vi "WSVCAP SHL Host LL Core.vi"(0 "Message In":string, 11 "error in":errorcluster, 12 "Log (T)":bool=TRUE, 13 "Function":T3) -> (3 "System":T1={"Settings"={"FPGA Resource Name"="", "I2C Slave Address"=20, "I2C Clock Rate (Hz)"=50000.0, "SPI Clock Rate (Hz)"=50000.0, "RFFE Slave Address"=20, "RFFE Clock Rate (Hz)"=50000.0, "Simulate FPGA"=TRUE, "C1 Cap DAC Default"=165, "C2 Cap DAC Default"=134, "C3 Cap DAC Default"=150}, "FPGA Resource"="", "Online"=FALSE, "I2C Wait Ticks"=0, "SPI Wait Ticks"=0, "RFFE Wait Ticks"=0} {"Settings"."C3 Cap DAC Default" format="0x%02x"; "Settings"."C2 Cap DAC Default" format="0x%02x"; "Settings"."C1 Cap DAC Default" format="0x%02x"; "Settings"."RFFE Clock Rate (Hz)" format="%.0f Hz"; "Settings"."RFFE Slave Address" format="0x%02x"; "Settings"."I2C Clock Rate (Hz)" format="%.0f Hz"; "Settings"."SPI Clock Rate (Hz)" format="%.0f Hz"; "Settings"."I2C Slave Address" format="0x%02x"}, 4 "Message Out":string, 15 "error out":errorcluster)   [LabVIEW 2012]
uses:
  Type Defs/WSVCAP SHL Function Enum.ctl
  Type Defs/WSVCAP SHL Core System Cluster.ctl
  Type Defs/WSVCAP SHL I2C Settings Cluster.ctl
  user.lib/Utilities/Type Defs/MISC IO Choice Enum.ctl
  Type Defs/WSVCAP SHL Top Level Control Operation Enum.ctl
  Type Defs/WSVCAP SHL Top Level Control Enum.ctl
  Type Defs/WSVCAP SHL Manager Operation Enum.ctl
  user.lib/Configuration Files/Type Defs/CFG File Operation Enum.ctl
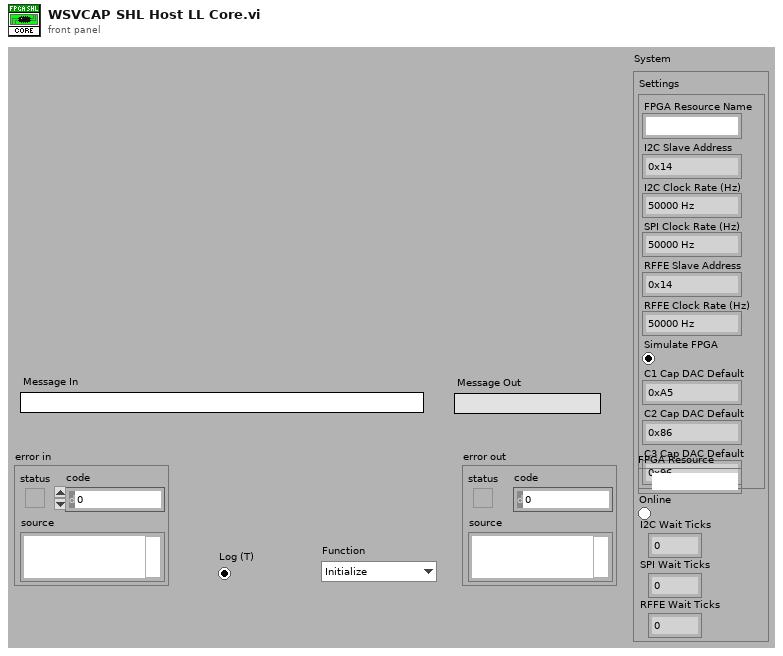
[diagram p1: front panel]
types:
  T1 = typedef "WSVCAP SHL Core System Cluster.ctl" = cluster{"Settings":T2, "FPGA Resource":tag, "Online":bool, "I2C Wait Ticks":u32, "SPI Wait Ticks":u32, "RFFE Wait Ticks":u32}
  T2 = typedef "WSVCAP SHL I2C Settings Cluster.ctl" = cluster{"FPGA Resource Name":string, "I2C Slave Address":u8, "I2C Clock Rate (Hz)":dbl, "SPI Clock Rate (Hz)":dbl, "RFFE Slave Address":u8, "RFFE Clock Rate (Hz)":dbl, "Simulate FPGA":bool, "C1 Cap DAC Default":u8, "C2 Cap DAC Default":u8, "C3 Cap DAC Default":u8}
  T3 = typedef "WSVCAP SHL Function Enum.ctl" = enum16{"Initialize", "Configure I2C", "Configure SPI", "Configure RFFE", "Write I2C", "Read I2C", "Write/Read SPI", "Start SPI Cycle", "Stop SPI Cycle", "Write RFFE", "Read RFFE", "Start RFFE Cycle", "Stop RFFE Cycle", "Get Status", "Close"}
  T4 = typedef "MISC IO Choice Enum.ctl" = enum16{"Read", "Write"}
  T5 = typedef "CFG File Operation Enum.ctl" = enum16{"Read", "Write", "Copy", "Edit"}
  T6 = typedef "WSVCAP SHL Manager Operation Enum.ctl" = enum16{"Initialize", "Close"}
  T7 = typedef "WSVCAP SHL Top Level Control Enum.ctl" = enum16{"Start", "Cmd", "Transaction", "Wait Ticks", "Socket Mask", "UUT Set", "Slave Address", "Sub Address", "Bytes to Write", "Bytes to Read", "Write Data", "Write Flag", "Read Data", "Read Flag", "Ack Read", "Read Status Flag", "Ack Read Status", "Status", "Cycle Count", "Stop Cycle", "Exit"}
  T8 = typedef "WSVCAP SHL Top Level Control Operation Enum.ctl" = enum16{"Initialize", "Set Control", "Read Control", "Close"}
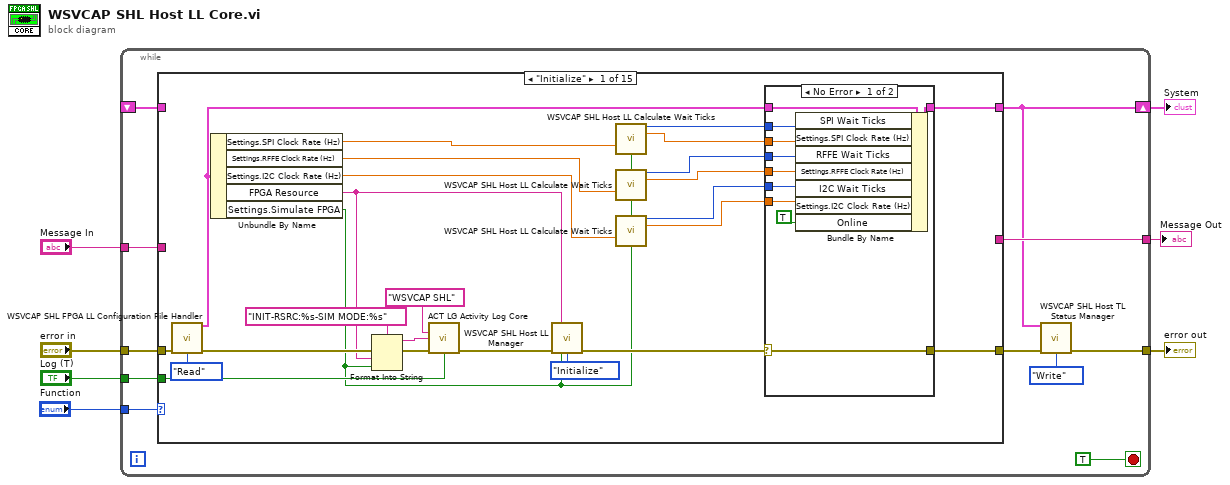
[diagram p0: block diagram]
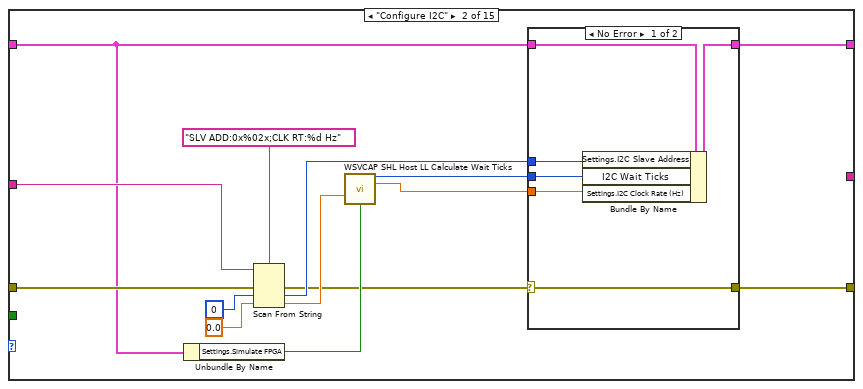
[diagram p3: hidden frame]
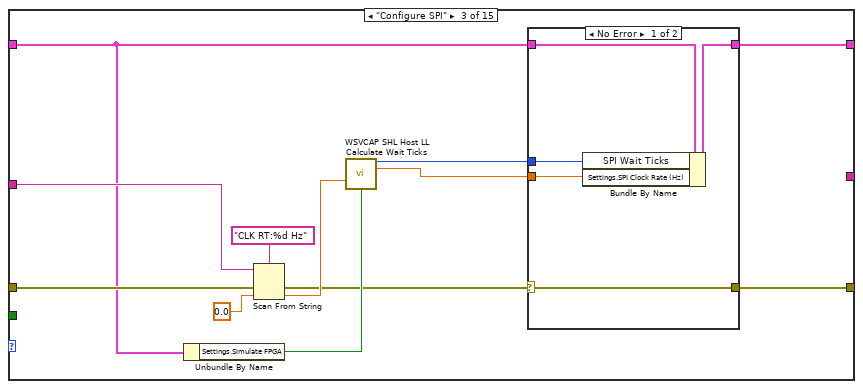
[diagram p5: hidden frame]
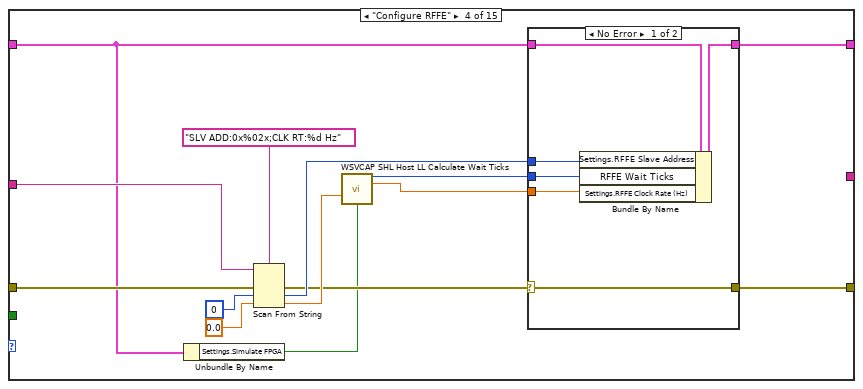
[diagram p7: hidden frame]
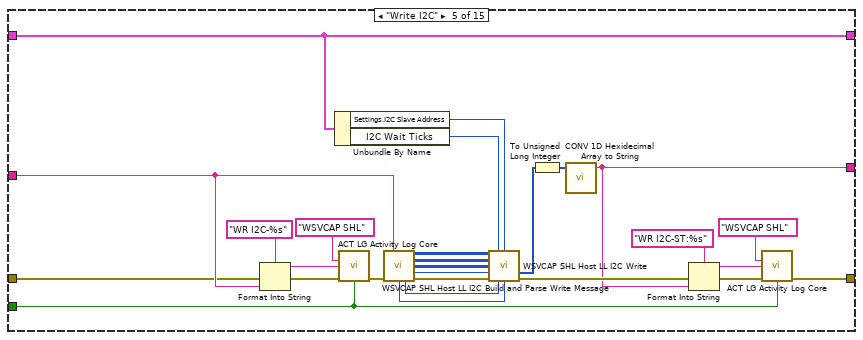
[diagram p9: hidden frame]
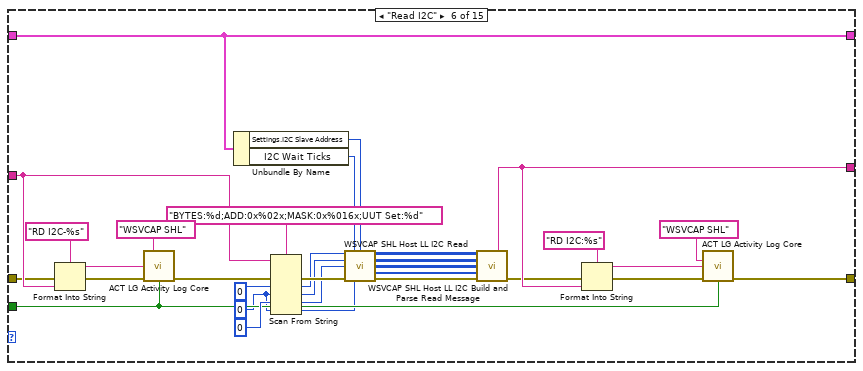
[diagram p10: hidden frame]
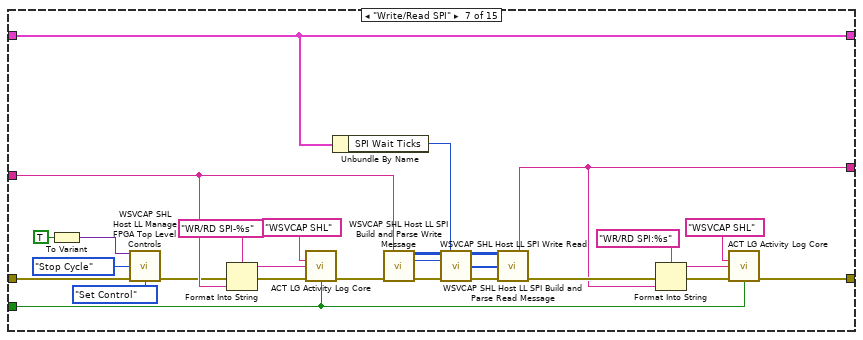
[diagram p11: hidden frame]
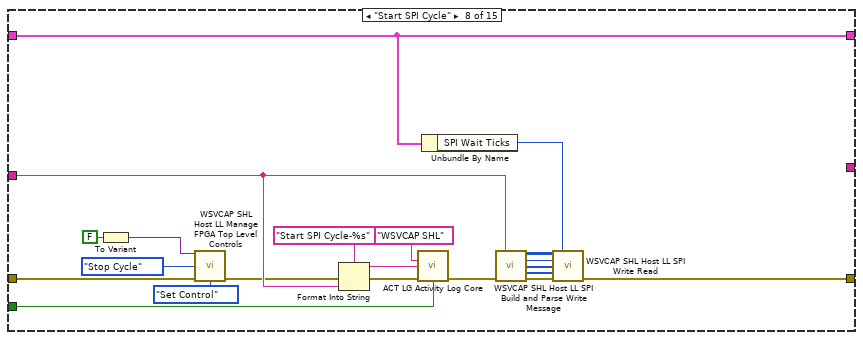
[diagram p12: hidden frame]
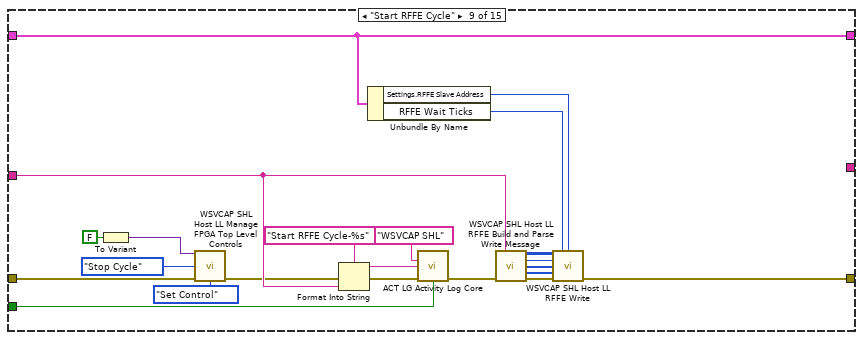
[diagram p13: hidden frame]
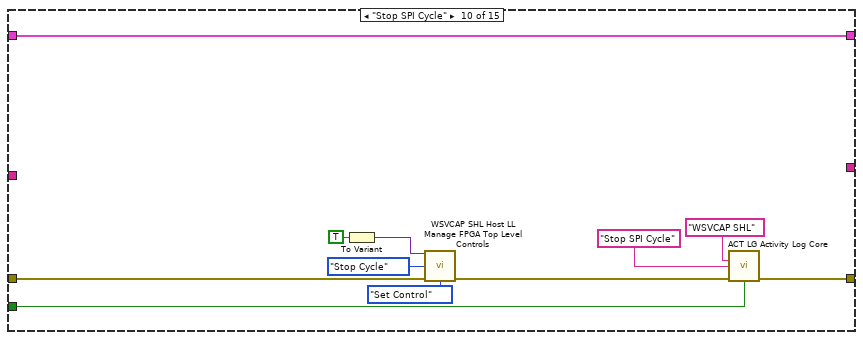
[diagram p14: hidden frame]
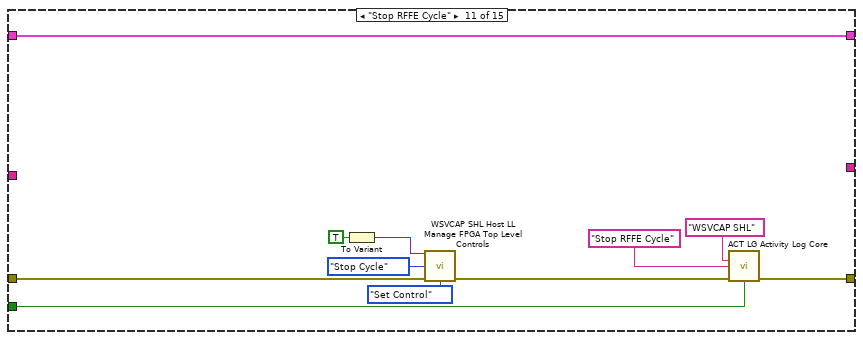
[diagram p15: hidden frame]
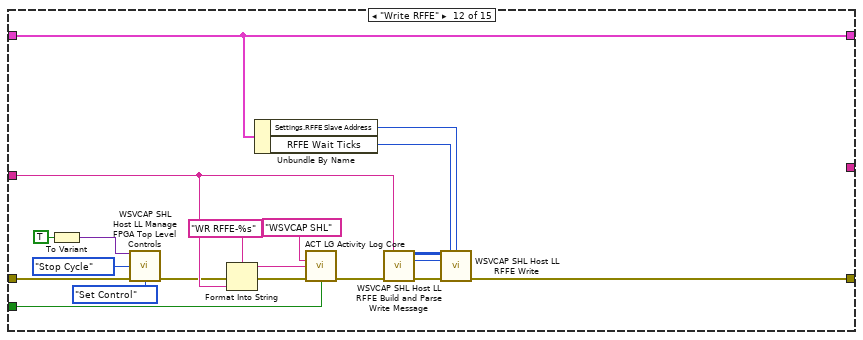
[diagram p16: hidden frame]
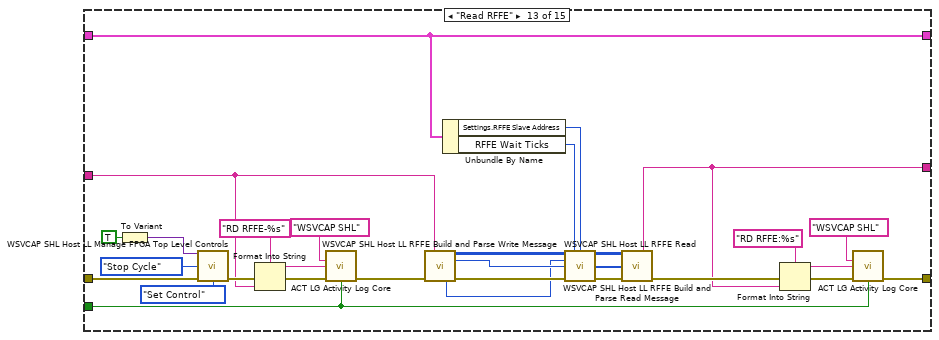
[diagram p17: hidden frame]
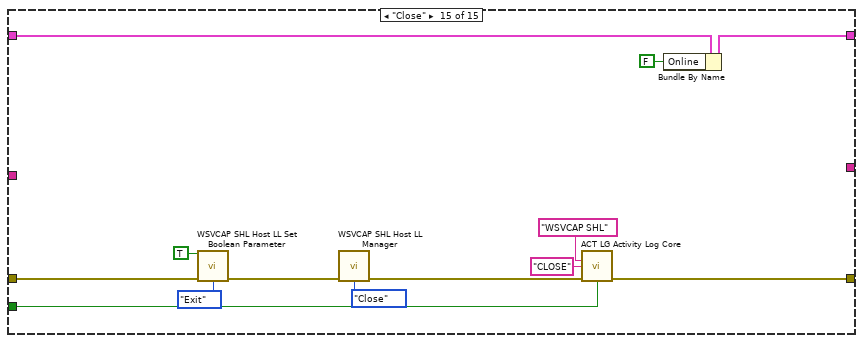
[diagram p19: hidden frame]
diagram:
  n1 = while {
    tunnel: "Function" -> [w17]
    tunnel: "error in" -> [w16]
    tunnel: "Message In" -> [w15]
    tunnel: [w11] -> w4
    shift-right: [w9] -> w3
    shift-left: _ -> [w14]
    tunnel: [w13] -> w2
    tunnel: "Log (T)" -> [w8]
    stop <- TRUE ("stop") stop-if-true
    n2 = case shown="\"Initialize\"" w17 {
      tunnel: w16 -> [w37 w67 w87 w108 w136 w159 w182 w209 w231 w250 w261 w277 w301 w321 w331]
      tunnel: w15 -> [_ w66 w86 w107 w137 w160 w188 w219 w241 _ _ w283 w294 _ _]
      tunnel: [w40 w68 w88 w109 w138 w156 w190 w217 w239 w257 w268 w272 w308 w321 w325] -> w12
      tunnel: [w41 w69 w89 w110 w124 w152 w179 w207 w229 w259 w270 w274 w299 w322 w334] -> w9
      tunnel: w14 -> [_ w62 w84 w103 w124 w152 w179 w207 w229 w259 w270 w274 w299 w322 w329]
      tunnel: [_ _ _ _ w128 w161 w189 _ _ _ _ _ w307 _ _] -> w13
      tunnel: w8 -> [w28 _ _ _ w125 w153 w187 w218 w240 w256 w267 w282 w306 _ w323]
      frame "Initialize" {
        n3 = call "WSVCAP SHL FPGA LL Configuration File Handler.vi"("Error In (no error)"=w37, "Operation"=CFG_File_Operation_Enum."Read") -> ("Object Cluster Out"=w42:T1, "Error Out"=w34:errorcluster)  [unwired: 11 in, 1 out]
        n4 = Unbundle By Name(w42) -> ("Settings.SPI Clock Rate (Hz)"=w22:dbl, "Settings.RFFE Clock Rate (Hz)"=w26:dbl, "Settings.I2C Clock Rate (Hz)"=w30:dbl, "FPGA Resource"=w31:tag, "Settings.Simulate FPGA"=w19:bool)
        n5 = Format Into String(format string="INIT-RSRC:%s-SIM MODE:%s", error in=w34, w31, w19) -> (resulting string=w35:string, error out=w33:errorcluster)  [unwired: 1 in]
        n6 = call "ACT LG Activity Log Core.vi"("Source"="WSVCAP SHL", "Log Line"=w35, "Error In (no error)"=w33, "Log (T)"=w28) -> ("Error Out"=w36:errorcluster)  [unwired: 10 in, 1 out]
        n7 = call "WSVCAP SHL Host LL Manager.vi"("FPGA Resource (Init Only)"=w31, "error in (no error)"=w36, "Simulate FPGA (Init Only)"=w19, "Operation"=WSVCAP_SHL_Manager_Operation_Enum."Initialize") -> ("error out"=w23:errorcluster)  [unwired: 11 in]
        n8 = call "WSVCAP SHL Host LL Calculate Wait Ticks.vi"("Clock Rate (Hz)"=w22, "Simulate FPGA"=w19) -> ("Wait Ticks"=w21:u32, "Actual Rate (Hz)"=w20:dbl)  [unwired: 12 in]
        n9 = call "WSVCAP SHL Host LL Calculate Wait Ticks.vi"("Clock Rate (Hz)"=w26, "Simulate FPGA"=w19) -> ("Wait Ticks"=w25:u32, "Actual Rate (Hz)"=w24:dbl)  [unwired: 12 in]
        n10 = call "WSVCAP SHL Host LL Calculate Wait Ticks.vi"("Clock Rate (Hz)"=w30, "Simulate FPGA"=w19) -> ("Wait Ticks"=w27:u32, "Actual Rate (Hz)"=w39:dbl)  [unwired: 12 in]
        n11 = case shown="No Error" w23 {
          selector: w23 -> [w51 w54]
          tunnel: w42 -> [w53 w55]
          tunnel: [w52 w55] -> w41
          tunnel: [w51 w54] -> w40
          tunnel: w39 -> [w50 _]
          tunnel: w27 -> [w48 _]
          tunnel: w25 -> [w47 _]
          tunnel: w24 -> [w46 _]
          tunnel: w21 -> [w45 _]
          tunnel: w20 -> [w44 _]
          frame No Error {
            n12 = Bundle By Name(cluster=w53, "SPI Wait Ticks"=w45, "Settings.SPI Clock Rate (Hz)"=w44, "RFFE Wait Ticks"=w47, "Settings.RFFE Clock Rate (Hz)"=w46, "I2C Wait Ticks"=w48, "Settings.I2C Clock Rate (Hz)"=w50, "Online"=TRUE) -> (w52:T1)
          }
          frame Error {
          }
        }
      }
      frame "Configure I2C" {
        n13 = Unbundle By Name(w62) -> ("Settings.Simulate FPGA"=w61:bool)
        n14 = Scan From String(format string="SLV ADD:0x%02x;CLK RT:%d Hz", input string=w66, error in=w67, default 1=u8 0 ("I2C_Slave Address"), default 2=0.0 ("Clock Rate (Hz)")) -> (error out=w56:errorcluster, output 1=w63:u8, output 2=w59:dbl)  [unwired: 1 in, 2 out]
        n15 = call "WSVCAP SHL Host LL Calculate Wait Ticks.vi"("Clock Rate (Hz)"=w59, "Simulate FPGA"=w61) -> ("Wait Ticks"=w57:u32, "Actual Rate (Hz)"=w58:dbl)  [unwired: 12 in]
        n16 = case shown="No Error" w56 {
          selector: w56 -> [w73 w76]
          tunnel: w62 -> [w75 w77]
          tunnel: [w74 w77] -> w69
          tunnel: [w73 w76] -> w68
          tunnel: w63 -> [w72 _]
          tunnel: w58 -> [w71 _]
          tunnel: w57 -> [w70 _]
          frame No Error {
            n17 = Bundle By Name(cluster=w75, "Settings.I2C Slave Address"=w72, "I2C Wait Ticks"=w70, "Settings.I2C Clock Rate (Hz)"=w71) -> (w74:T1)
          }
          frame Error {
          }
        }
      }
      frame "Configure SPI" {
        n18 = Unbundle By Name(w84) -> ("Settings.Simulate FPGA"=w79:bool)
        n19 = Scan From String(format string="CLK RT:%d Hz", input string=w86, error in=w87, default 1=0.0 ("Clock Rate (Hz)")) -> (error out=w78:errorcluster, output 1=w82:dbl)  [unwired: 1 in, 2 out]
        n20 = call "WSVCAP SHL Host LL Calculate Wait Ticks.vi"("Clock Rate (Hz)"=w82, "Simulate FPGA"=w79) -> ("Wait Ticks"=w81:u32, "Actual Rate (Hz)"=w80:dbl)  [unwired: 12 in]
        n21 = case shown="No Error" w78 {
          selector: w78 -> [w92 w95]
          tunnel: w84 -> [w94 w96]
          tunnel: [w93 w96] -> w89
          tunnel: [w92 w95] -> w88
          tunnel: w80 -> [w91 _]
          tunnel: w81 -> [w90 _]
          frame No Error {
            n22 = Bundle By Name(cluster=w94, "SPI Wait Ticks"=w90, "Settings.SPI Clock Rate (Hz)"=w91) -> (w93:T1)
          }
          frame Error {
          }
        }
      }
      frame "Configure RFFE" {
        n23 = Unbundle By Name(w103) -> ("Settings.Simulate FPGA"=w97:bool)
        n24 = Scan From String(format string="SLV ADD:0x%02x;CLK RT:%d Hz", input string=w107, error in=w108, default 1=u8 0 ("I2C_Slave Address"), default 2=0.0 ("Clock Rate (Hz)")) -> (error out=w98:errorcluster, output 1=w104:u8, output 2=w101:dbl)  [unwired: 1 in, 2 out]
        n25 = call "WSVCAP SHL Host LL Calculate Wait Ticks.vi"("Clock Rate (Hz)"=w101, "Simulate FPGA"=w97) -> ("Wait Ticks"=w100:u32, "Actual Rate (Hz)"=w99:dbl)  [unwired: 12 in]
        n26 = case shown="No Error" w98 {
          selector: w98 -> [w114 w117]
          tunnel: w103 -> [w116 w118]
          tunnel: [w115 w118] -> w110
          tunnel: [w114 w117] -> w109
          tunnel: w104 -> [w113 _]
          tunnel: w99 -> [w112 _]
          tunnel: w100 -> [w111 _]
          frame No Error {
            n27 = Bundle By Name(cluster=w116, "Settings.RFFE Slave Address"=w113, "RFFE Wait Ticks"=w111, "Settings.RFFE Clock Rate (Hz)"=w112) -> (w115:T1)
          }
          frame Error {
          }
        }
      }
      frame "Write I2C" {
        n28 = Format Into String(format string="WR I2C-%s", error in=w136, w137) -> (resulting string=w133:string, error out=w135:errorcluster)  [unwired: 1 in]
        n29 = Unbundle By Name(w124) -> ("Settings.I2C Slave Address"=w120:u8, "I2C Wait Ticks"=w123:u32)
        n30 = call "ACT LG Activity Log Core.vi"("Source"="WSVCAP SHL", "Log Line"=w133, "Error In (no error)"=w135, "Log (T)"=w125) -> ("Error Out"=w140:errorcluster)  [unwired: 10 in, 1 out]
        n31 = call "WSVCAP SHL Host LL I2C Build and Parse Write Message.vi"("Message In"=w137, "error in"=w140) -> ("C1 Write Data Out [DUT Ordered]"=w144:u8[][], "C2 Write Data Out [DUT Ordered]"=w142:u8[][], "C3 Write Data Out [DUT Ordered]"=w122:u8[][], "Socket Mask [U64] Out"=w143:u64, "UUT Set (0/1) Out"=w119:u8, "Sub Address Out"=w121:u8, "error out"=w145:errorcluster)  [unwired: 6 in, 1 out]
        n32 = call "WSVCAP SHL Host LL I2C Write.vi"("C1 Data Out [DUT Ordered]"=w144, "Wait Ticks"=w123, "Slave Address"=w120, "C2 Data Out [DUT Ordered]"=w142, "C3 Data Out [DUT Ordered]"=w122, "Socket Mask [U64]"=w143, "error in"=w145, "Sub Address"=w121, "UUT Set (0/1)"=w119) -> ("Status"=w130:u8[], "error out"=w132:errorcluster)  [unwired: 5 in]
        n33 = To Unsigned Long Integer(number=w130) -> (unsigned 32bit integer=w129:u32[])
        n34 = call "CONV 1D Hexidecimal Array to String.vi"("1-D Hexidecimal"=w129) -> ("String"=w128:string)  [unwired: 8 in]
        n35 = Format Into String(format string="WR I2C-ST:%s", error in=w132, w128) -> (resulting string=w126:string, error out=w131:errorcluster)  [unwired: 1 in]
        n36 = call "ACT LG Activity Log Core.vi"("Source"="WSVCAP SHL", "Log Line"=w126, "Error In (no error)"=w131, "Log (T)"=w125) -> ("Error Out"=w138:errorcluster)  [unwired: 10 in, 1 out]
      }
      frame "Read I2C" {
        w147 = u8 0 ("Sub Address [U8]")
        n37 = Format Into String(format string="RD I2C-%s", error in=w159, w160) -> (resulting string=w165:string, error out=w167:errorcluster)  [unwired: 1 in]
        n38 = call "ACT LG Activity Log Core.vi"("Source"="WSVCAP SHL", "Log Line"=w165, "Error In (no error)"=w167, "Log (T)"=w153) -> ("Error Out"=w158:errorcluster)  [unwired: 10 in, 1 out]
        n39 = Unbundle By Name(w152) -> ("Settings.I2C Slave Address"=w148:u8, "I2C Wait Ticks"=w151:u32)
        n40 = Scan From String(format string="BYTES:%d;ADD:0x%02x;MASK:0x%016x;UUT Set:%d", input string=w160, error in=w158, default 1=u8 0 ("Bytes to Read"), default 2=w147, default 3=u64 0 ("Socket Mask [U32]"), default 4=w147) -> (error out=w177:errorcluster, output 1=w174:u8, output 2=w172:u8, output 3=w173:u64, output 4=w146:u8)  [unwired: 1 in, 2 out]
        n41 = call "WSVCAP SHL Host LL I2C Read.vi"("Bytes to Read"=w174, "Wait Ticks"=w151, "Slave Address"=w148, "Sub Address [U8]"=w172, "Socket Mask [U64]"=w173, "error in"=w177, "UUT Set (0/1)"=w146) -> ("C1:1-18 Read Data [DUT Ordered]"=w170:u8[][], "C2:1-18 Read Data [DUT Ordered]"=w169:u8[][], "C3:1-18 Read Data [DUT Ordered]"=w150:u8[][], "Status"=w149:u8[], "error out"=w171:errorcluster)  [unwired: 4 in]
        n42 = call "WSVCAP SHL Host LL I2C Build and Parse Read Message.vi"("C1 Read Data In"=w170, "C2 Read Data"=w169, "C3 Read Data"=w150, "Status In"=w149, "error in"=w171) -> ("Message Out"=w161:string, "error out"=w157:errorcluster)  [unwired: 5 in, 4 out]
        n43 = Format Into String(format string="RD I2C:%s", error in=w157, w161) -> (resulting string=w162:string, error out=w164:errorcluster)  [unwired: 1 in]
        n44 = call "ACT LG Activity Log Core.vi"("Source"="WSVCAP SHL", "Log Line"=w162, "Error In (no error)"=w164, "Log (T)"=w153) -> ("Error Out"=w156:errorcluster)  [unwired: 10 in, 1 out]
      }
      frame "Write/Read SPI" {
        n45 = To Variant(anything=TRUE ("Cycle (F:Write/Read - T:Write Only - No Read)")) -> (Variant=w184:variant)
        n46 = call "WSVCAP SHL Host LL Manage FPGA Top Level Controls.vi"("Value In"=w184, "FPGA Top Level Control"=WSVCAP_SHL_Top_Level_Control_Enum."Stop Cycle", "error in (no error)"=w182, "Operation"=WSVCAP_SHL_Top_Level_Control_Operation_Enum."Set Control") -> ("error out"=w181:errorcluster)  [unwired: 10 in, 1 out]
        n47 = Format Into String(format string="WR/RD SPI-%s", error in=w181, w188) -> (resulting string=w196:string, error out=w198:errorcluster)  [unwired: 1 in]
        n48 = call "ACT LG Activity Log Core.vi"("Source"="WSVCAP SHL", "Log Line"=w196, "Error In (no error)"=w198, "Log (T)"=w187) -> ("Error Out"=w192:errorcluster)  [unwired: 10 in, 1 out]
        n49 = Unbundle By Name(w179) -> ("SPI Wait Ticks"=w178:u32)
        n50 = call "WSVCAP SHL Host LL SPI Build and Parse Write Message.vi"("Message In"=w188, "error in"=w192) -> ("Write Data Out [DUT Ordered]"=w204:u8[][], "Socket Mask [U16] Out"=w180:u16, "error out"=w205:errorcluster)  [unwired: 8 in, 3 out]
        n51 = call "WSVCAP SHL Host LL SPI Write Read.vi"("SPI Data [DUT Ordered]"=w204, "Wait Ticks"=w178, "Socket Mask"=w180, "error in"=w205) -> ("SPI Read Data [DUT Ordered]"=w202:u8[][], "Status"=w201:u8[], "error out"=w203:errorcluster)  [unwired: 9 in]
        n52 = call "WSVCAP SHL Host LL SPI Build and Parse Read Message.vi"("Write Data In"=w202, "Status In"=w201, "error in"=w203) -> ("Message Out"=w189:string, "error out"=w191:errorcluster)  [unwired: 9 in, 2 out]
        n53 = Format Into String(format string="WR/RD SPI:%s", error in=w191, w189) -> (resulting string=w193:string, error out=w195:errorcluster)  [unwired: 1 in]
        n54 = call "ACT LG Activity Log Core.vi"("Source"="WSVCAP SHL", "Log Line"=w193, "Error In (no error)"=w195, "Log (T)"=w187) -> ("Error Out"=w190:errorcluster)  [unwired: 10 in, 1 out]
      }
      frame "Start SPI Cycle" {
        n55 = To Variant(anything=FALSE ("Cycle (F:Write/Read - T:Write Only - No Read)")) -> (Variant=w214:variant)
        n56 = call "WSVCAP SHL Host LL Manage FPGA Top Level Controls.vi"("Value In"=w214, "FPGA Top Level Control"=WSVCAP_SHL_Top_Level_Control_Enum."Stop Cycle", "error in (no error)"=w209, "Operation"=WSVCAP_SHL_Top_Level_Control_Operation_Enum."Set Control") -> ("error out"=w208:errorcluster)  [unwired: 10 in, 1 out]
        n57 = Format Into String(format string="Start SPI Cycle-%s", error in=w208, w219) -> (resulting string=w221:string, error out=w223:errorcluster)  [unwired: 1 in]
        n58 = call "ACT LG Activity Log Core.vi"("Source"="WSVCAP SHL", "Log Line"=w221, "Error In (no error)"=w223, "Log (T)"=w218) -> ("Error Out"=w220:errorcluster)  [unwired: 10 in, 1 out]
        n59 = Unbundle By Name(w207) -> ("SPI Wait Ticks"=w206:u32)
        n60 = call "WSVCAP SHL Host LL SPI Build and Parse Write Message.vi"("Message In"=w219, "error in"=w220) -> ("Write Data Out [DUT Ordered]"=w225:u8[][], "Socket Mask [U16] Out"=w212:u16, "Cycle CMD Lengths Out (bits)"=w211:u8[], "Cycle CMD Delay Out (ticks)"=w210:u32[], "error out"=w226:errorcluster)  [unwired: 8 in, 1 out]
        n61 = call "WSVCAP SHL Host LL SPI Write Read.vi"("SPI Data [DUT Ordered]"=w225, "Wait Ticks"=w206, "Socket Mask"=w212, "Cycle CMD Lengths Out (bits)"=w211, "Cycle CMD Delay Out (ticks)"=w210, "error in"=w226) -> ("error out"=w217:errorcluster)  [unwired: 7 in, 2 out]
      }
      frame "Start RFFE Cycle" {
        n62 = To Variant(anything=FALSE ("Cycle (F:Write/Read - T:Write Only - No Read)")) -> (Variant=w236:variant)
        n63 = call "WSVCAP SHL Host LL Manage FPGA Top Level Controls.vi"("Value In"=w236, "FPGA Top Level Control"=WSVCAP_SHL_Top_Level_Control_Enum."Stop Cycle", "error in (no error)"=w231, "Operation"=WSVCAP_SHL_Top_Level_Control_Operation_Enum."Set Control") -> ("error out"=w230:errorcluster)  [unwired: 10 in, 1 out]
        n64 = Format Into String(format string="Start RFFE Cycle-%s", error in=w230, w241) -> (resulting string=w243:string, error out=w245:errorcluster)  [unwired: 1 in]
        n65 = Unbundle By Name(w229) -> ("Settings.RFFE Slave Address"=w227:u8, "RFFE Wait Ticks"=w228:u32)
        n66 = call "ACT LG Activity Log Core.vi"("Source"="WSVCAP SHL", "Log Line"=w243, "Error In (no error)"=w245, "Log (T)"=w240) -> ("Error Out"=w242:errorcluster)  [unwired: 10 in, 1 out]
        n67 = call "WSVCAP SHL Host LL RFFE Build and Parse Write Message.vi"("Message In"=w241, "error in"=w242) -> ("Write Data Out [DUT Ordered]"=w247:u8[][], "Socket Mask [U16] Out"=w234:u64, "Cycle CMD Lengths Out (bits)"=w233:u8[], "Cycle CMD Delay Out (ticks)"=w232:u32[], "error out"=w248:errorcluster)  [unwired: 7 in, 2 out]
        n68 = call "WSVCAP SHL Host LL RFFE Write.vi"("RTFFE Data [DUT Ordered]"=w247, "Wait Ticks"=w228, "Slave Address"=w227, "Socket Mask"=w234, "Cycle CMD Lengths Out (bits)"=w233, "Cycle CMD Delay Out (ticks)"=w232, "error in"=w248) -> ("error out"=w239:errorcluster)  [unwired: 7 in, 1 out]
      }
      frame "Stop SPI Cycle" {
        n69 = To Variant(anything=TRUE ("Cycle (F:Write/Read - T:Write Only - No Read)")) -> (Variant=w252:variant)
        n70 = call "WSVCAP SHL Host LL Manage FPGA Top Level Controls.vi"("Value In"=w252, "FPGA Top Level Control"=WSVCAP_SHL_Top_Level_Control_Enum."Stop Cycle", "error in (no error)"=w250, "Operation"=WSVCAP_SHL_Top_Level_Control_Operation_Enum."Set Control") -> ("error out"=w249:errorcluster)  [unwired: 10 in, 1 out]
        n71 = call "ACT LG Activity Log Core.vi"("Source"="WSVCAP SHL", "Log Line"="Stop SPI Cycle" ("format string"), "Error In (no error)"=w249, "Log (T)"=w256) -> ("Error Out"=w257:errorcluster)  [unwired: 10 in, 1 out]
      }
      frame "Stop RFFE Cycle" {
        n72 = To Variant(anything=TRUE ("Cycle (F:Write/Read - T:Write Only - No Read)")) -> (Variant=w263:variant)
        n73 = call "WSVCAP SHL Host LL Manage FPGA Top Level Controls.vi"("Value In"=w263, "FPGA Top Level Control"=WSVCAP_SHL_Top_Level_Control_Enum."Stop Cycle", "error in (no error)"=w261, "Operation"=WSVCAP_SHL_Top_Level_Control_Operation_Enum."Set Control") -> ("error out"=w260:errorcluster)  [unwired: 10 in, 1 out]
        n74 = call "ACT LG Activity Log Core.vi"("Source"="WSVCAP SHL", "Log Line"="Stop RFFE Cycle" ("format string"), "Error In (no error)"=w260, "Log (T)"=w267) -> ("Error Out"=w268:errorcluster)  [unwired: 10 in, 1 out]
      }
      frame "Write RFFE" {
        n75 = To Variant(anything=TRUE ("Cycle (F:Write/Read - T:Write Only - No Read)")) -> (Variant=w279:variant)
        n76 = call "WSVCAP SHL Host LL Manage FPGA Top Level Controls.vi"("Value In"=w279, "FPGA Top Level Control"=WSVCAP_SHL_Top_Level_Control_Enum."Stop Cycle", "error in (no error)"=w277, "Operation"=WSVCAP_SHL_Top_Level_Control_Operation_Enum."Set Control") -> ("error out"=w276:errorcluster)  [unwired: 10 in, 1 out]
        n77 = Format Into String(format string="WR RFFE-%s", error in=w276, w283) -> (resulting string=w285:string, error out=w287:errorcluster)  [unwired: 1 in]
        n78 = Unbundle By Name(w274) -> ("Settings.RFFE Slave Address"=w271:u8, "RFFE Wait Ticks"=w273:u32)
        n79 = call "ACT LG Activity Log Core.vi"("Source"="WSVCAP SHL", "Log Line"=w285, "Error In (no error)"=w287, "Log (T)"=w282) -> ("Error Out"=w284:errorcluster)  [unwired: 10 in, 1 out]
        n80 = call "WSVCAP SHL Host LL RFFE Build and Parse Write Message.vi"("Message In"=w283, "error in"=w284) -> ("Write Data Out [DUT Ordered]"=w289:u8[][], "Socket Mask [U16] Out"=w275:u64, "error out"=w290:errorcluster)  [unwired: 7 in, 4 out]
        n81 = call "WSVCAP SHL Host LL RFFE Write.vi"("RTFFE Data [DUT Ordered]"=w289, "Wait Ticks"=w273, "Slave Address"=w271, "Socket Mask"=w275, "error in"=w290) -> ("error out"=w272:errorcluster)  [unwired: 9 in, 1 out]
      }
      frame "Read RFFE" {
        n82 = To Variant(anything=TRUE ("Cycle (F:Write/Read - T:Write Only - No Read)")) -> (Variant=w303:variant)
        n83 = call "WSVCAP SHL Host LL Manage FPGA Top Level Controls.vi"("Value In"=w303, "FPGA Top Level Control"=WSVCAP_SHL_Top_Level_Control_Enum."Stop Cycle", "error in (no error)"=w301, "Operation"=WSVCAP_SHL_Top_Level_Control_Operation_Enum."Set Control") -> ("error out"=w300:errorcluster)  [unwired: 10 in, 1 out]
        n84 = Format Into String(format string="RD RFFE-%s", error in=w300, w294) -> (resulting string=w313:string, error out=w315:errorcluster)  [unwired: 1 in]
        n85 = call "ACT LG Activity Log Core.vi"("Source"="WSVCAP SHL", "Log Line"=w313, "Error In (no error)"=w315, "Log (T)"=w306) -> ("Error Out"=w296:errorcluster)  [unwired: 10 in, 1 out]
        n86 = call "WSVCAP SHL Host LL RFFE Build and Parse Write Message.vi"("Message In"=w294, "error in"=w296) -> ("Write Data Out [DUT Ordered]"=w293:u8[][], "Socket Mask [U16] Out"=w292:u64, "Byte Count"=w291:u8, "error out"=w295:errorcluster)  [unwired: 7 in, 3 out]
        n87 = Unbundle By Name(w299) -> ("Settings.RFFE Slave Address"=w297:u8, "RFFE Wait Ticks"=w298:u32)
        n88 = call "WSVCAP SHL Host LL RFFE Read.vi"("RFFE Data [DUT Ordered]"=w293, "Wait Ticks"=w298, "Slave Address"=w297, "Bytes to Read"=w291, "Socket Mask [U64]"=w292, "error in"=w295) -> ("RFFE Read Data [DUT Ordered]"=w319:u8[][], "Status"=w318:u8[], "error out"=w320:errorcluster)  [unwired: 7 in]
        n89 = call "WSVCAP SHL Host LL RFFE Build and Parse Read Message.vi"("Write Data In"=w319, "Status In"=w318, "error in"=w320) -> ("Message Out"=w307:string, "error out"=w309:errorcluster)  [unwired: 9 in, 2 out]
        n90 = Format Into String(format string="RD RFFE:%s", error in=w309, w307) -> (resulting string=w310:string, error out=w312:errorcluster)  [unwired: 1 in]
        n91 = call "ACT LG Activity Log Core.vi"("Source"="WSVCAP SHL", "Log Line"=w310, "Error In (no error)"=w312, "Log (T)"=w306) -> ("Error Out"=w308:errorcluster)  [unwired: 10 in, 1 out]
      }
      frame "Get Status" {
      }
      frame "Close" {
        n92 = call "WSVCAP SHL Host LL Set Boolean Parameter.vi"("Boolean In"=TRUE ("Start"), "error in (no error)"=w331, "FPGA Top Level Control"=WSVCAP_SHL_Top_Level_Control_Enum."Exit") -> ("error out"=w330:errorcluster)  [unwired: 12 in]
        n93 = call "WSVCAP SHL Host LL Manager.vi"("error in (no error)"=w330, "Operation"=WSVCAP_SHL_Manager_Operation_Enum."Close") -> ("error out"=w326:errorcluster)  [unwired: 13 in]
        n94 = call "ACT LG Activity Log Core.vi"("Source"="WSVCAP SHL", "Log Line"="CLOSE", "Error In (no error)"=w326, "Log (T)"=w323) -> ("Error Out"=w325:errorcluster)  [unwired: 10 in, 1 out]
        n95 = Bundle By Name(cluster=w329, "Online"=FALSE) -> (w334:T1)
      }
    }
    n96 = call "WSVCAP SHL Host TL Status Manager.vi"("System In"=w9, "error in"=w12, "Operation (Read)"=MISC_IO_Choice_Enum."Write") -> ("error out"=w11:errorcluster)  [unwired: 11 in, 1 out]
  }
  "error out" <- w4
  "Message Out" <- w2
  "System" <- w3
